vi "Configure Trigger (Delay Trigger Characteristics).vi"(0 "VISA resource name":refnum<visa-resource-name>, 1 "Trigger Source (1: Channel 1)":u16(ring)=1 items=["Channel 1"=1, "Channel 2"=2, "Channel 3"=3, "Channel 4"=4, "Digital 0"=13, "Digital 1"=14, "Digital 2"=15, "Digital 3"=16, "Digital 4"=17, "Digital 5"=18, "Digital 6"=19, "Digital 7"=20, "Digital 8"=21, "Digital 9"=22, "Digital 10"=23, "Digital 11"=24, "Digital 12"=25, "Digital 13"=26, "Digital 14"=27, "Digital 15"=28], 2 "Trigger Slope (0: Positive)":u16(ring) items=["Positive", "Negative"], 3 "Trigger Level (0.0 V)":dbl, 5 "Arm Source (1: Channel 1)":u16(ring)=1 items=["Channel 1"=1, "Channel 2"=2, "Channel 3"=3, "Channel 4"=4, "Digital 0"=13, "Digital 1"=14, "Digital 2"=15, "Digital 3"=16, "Digital 4"=17, "Digital 5"=18, "Digital 6"=19, "Digital 7"=20, "Digital 8"=21, "Digital 9"=22, "Digital 10"=23, "Digital 11"=24, "Digital 12"=25, "Digital 13"=26, "Digital 14"=27, "Digital 15"=28], 7 "Arm Slope (0: Positive)":u16(ring) items=["Positive", "Negative"], 9 "Arm Level (0.0 V)":dbl, 11 "error in (no error)":errorcluster) -> (4 "VISA resource name out":refnum<visa-resource-name>, 15 "error out":errorcluster)   [LabVIEW 2012, in "Agilent 8000 Series.lvlib"]
doc: "Configures the delay Source. It configures the Arm Source, Arm Slope, Arm level,Trigger Source, Trigger Slope, Trigger level."
uses:
  Agilent 8000 Series.lvlib
panel:
  # "Arm On"
  # "Trigger On"
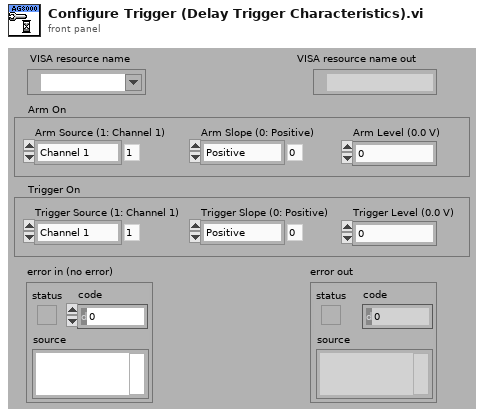
[diagram p1: front panel]
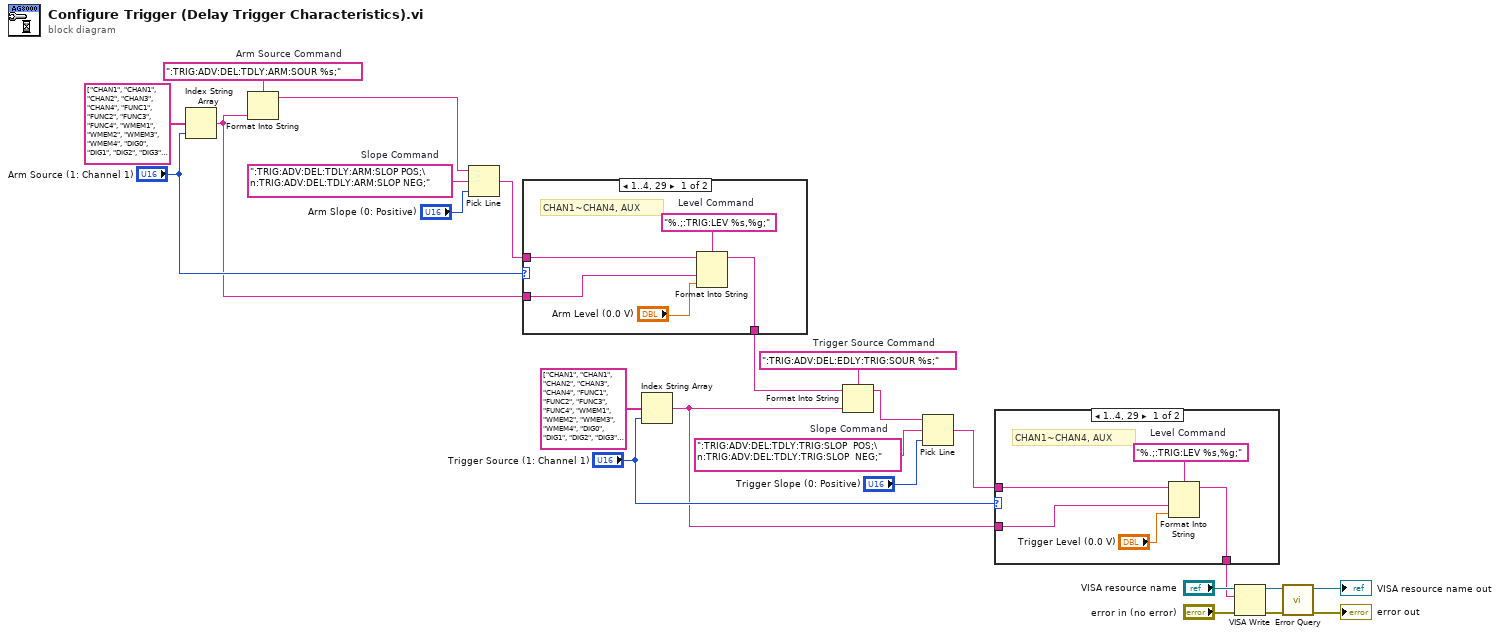
[diagram p0: block diagram]
diagram:
  w6 = ":TRIG:ADV:DEL:TDLY:TRIG:SLOP  POS;\n:TRIG:ADV:DEL:TDLY:TRIG:SLOP  NEG;"  # Slope Command
  w8 = ":TRIG:ADV:DEL:EDLY:TRIG:SOUR %s;"  # Trigger Source Command
  w15 = ":TRIG:ADV:DEL:TDLY:ARM:SLOP POS;\n:TRIG:ADV:DEL:TDLY:ARM:SLOP NEG;"  # Slope Command
  w17 = ":TRIG:ADV:DEL:TDLY:ARM:SOUR %s;"  # Arm Source Command
  n1 = Index String Array(1:"Arm Source (1: Channel 1)", 2:string[] ["CHAN1", "CHAN1", "CHAN2", "CHAN3", "CHAN4", "FUNC1", "FUNC2", "FUNC3", "FUNC4", "WMEM1", "WMEM2", "WMEM3", "WMEM4", "DIG0", "DIG1", "DIG2", "DIG3", "DIG4", "DIG5", "DIG6", "DIG7", "DIG8", "DIG9", "DIG10", "DIG11", "DIG12", "DIG13", "DIG14", "DIG15", "AUX", "LINE"]) -> (0:w12:string)  [unwired: 1 in]
  n2 = Format Into String(format string=w17, w12) -> (resulting string=w13:string)  [unwired: 2 in, 1 out]
  n3 = Pick Line(string ("")=w13, multi-line string=w15, line index="Arm Slope (0: Positive)") -> (output string=w11:string)
  n4 = case shown="1..4, 29" "Arm Source (1: Channel 1)" {
    tunnel: [w28 w30] -> w9
    tunnel: w12 -> [w27 _]
    tunnel: w11 -> [w26 w30]
    frame 1..4, 29 {
      w29 = "%.;:TRIG:LEV %s,%g;"  # Level Command
      # "CHAN1~CHAN4, AUX"
      n5 = Format Into String(format string=w29, initial string=w26, w27, "Arm Level (0.0 V)") -> (resulting string=w28:string)  [unwired: 1 in, 1 out]
    }
    frame Default {
      # "DIG0~DIG15"
    }
  }
  n6 = Index String Array(1:"Trigger Source (1: Channel 1)", 2:string[] ["CHAN1", "CHAN1", "CHAN2", "CHAN3", "CHAN4", "FUNC1", "FUNC2", "FUNC3", "FUNC4", "WMEM1", "WMEM2", "WMEM3", "WMEM4", "DIG0", "DIG1", "DIG2", "DIG3", "DIG4", "DIG5", "DIG6", "DIG7", "DIG8", "DIG9", "DIG10", "DIG11", "DIG12", "DIG13", "DIG14", "DIG15", "AUX", "LINE"]) -> (0:w3:string)  [unwired: 1 in]
  n7 = Format Into String(format string=w8, initial string=w9, w3) -> (resulting string=w7:string)  [unwired: 1 in, 1 out]
  n8 = Pick Line(string ("")=w7, multi-line string=w6, line index="Trigger Slope (0: Positive)") -> (output string=w2:string)
  n9 = case shown="1..4, 29" "Trigger Source (1: Channel 1)" {
    tunnel: [w34 w36] -> w1
    tunnel: w3 -> [w33 _]
    tunnel: w2 -> [w32 w36]
    frame 1..4, 29 {
      w35 = "%.;:TRIG:LEV %s,%g;"  # Level Command
      # "CHAN1~CHAN4, AUX"
      n10 = Format Into String(format string=w35, initial string=w32, w33, "Trigger Level (0.0 V)") -> (resulting string=w34:string)  [unwired: 1 in, 1 out]
    }
    frame Default {
      # "DIG0~DIG15"
    }
  }
  n11 = VISA Write(VISA resource name="VISA resource name", write buffer=w1, error in (no error)="error in (no error)") -> (VISA resource name out=w20:refnum<visa-resource-name>, error out=w19:errorcluster)  [unwired: 1 out]
  n12 = call "Error Query.vi"("error in (no error)"=w19, "VISA resource name"=w20) -> ("error out"=→"error out":errorcluster, "VISA resource name out"=→"VISA resource name out":refnum<visa-resource-name>)  [unwired: 6 in, 2 out]
